vi "SQL查询.vi"(7 "condition":string, 9 "columns":string[](array[string]), 10 "table输入":string(combo), 11 "database":string(combo)) -> (0 "error out":errorcluster, 1 "拆分数据":bool, 2 "columns输出":string[](array[string]), 3 "data":string[][](table))   [LabVIEW 2016, in "数据传输系统-03.lvlib"]
uses:
  <vilib>/Utility/sysdir.llb/System Directory Type.ctl
  <vilib>/addons/database/Connection.llb/DB Tools Open Connec (String).vi
  <vilib>/addons/database/_DB Variant To Data/Database Variant To Data.xnode
  <vilib>/addons/database/NI_Database_API.lvlib
panel:
  out "元素":string
  out "子数组":string[](array[string])
  in  "error in (no error)":errorcluster
  # "时间 > #2021/01/15 08:00:00#and 时间 < #2021/04/15 08:00:00# order by 时间 asc"
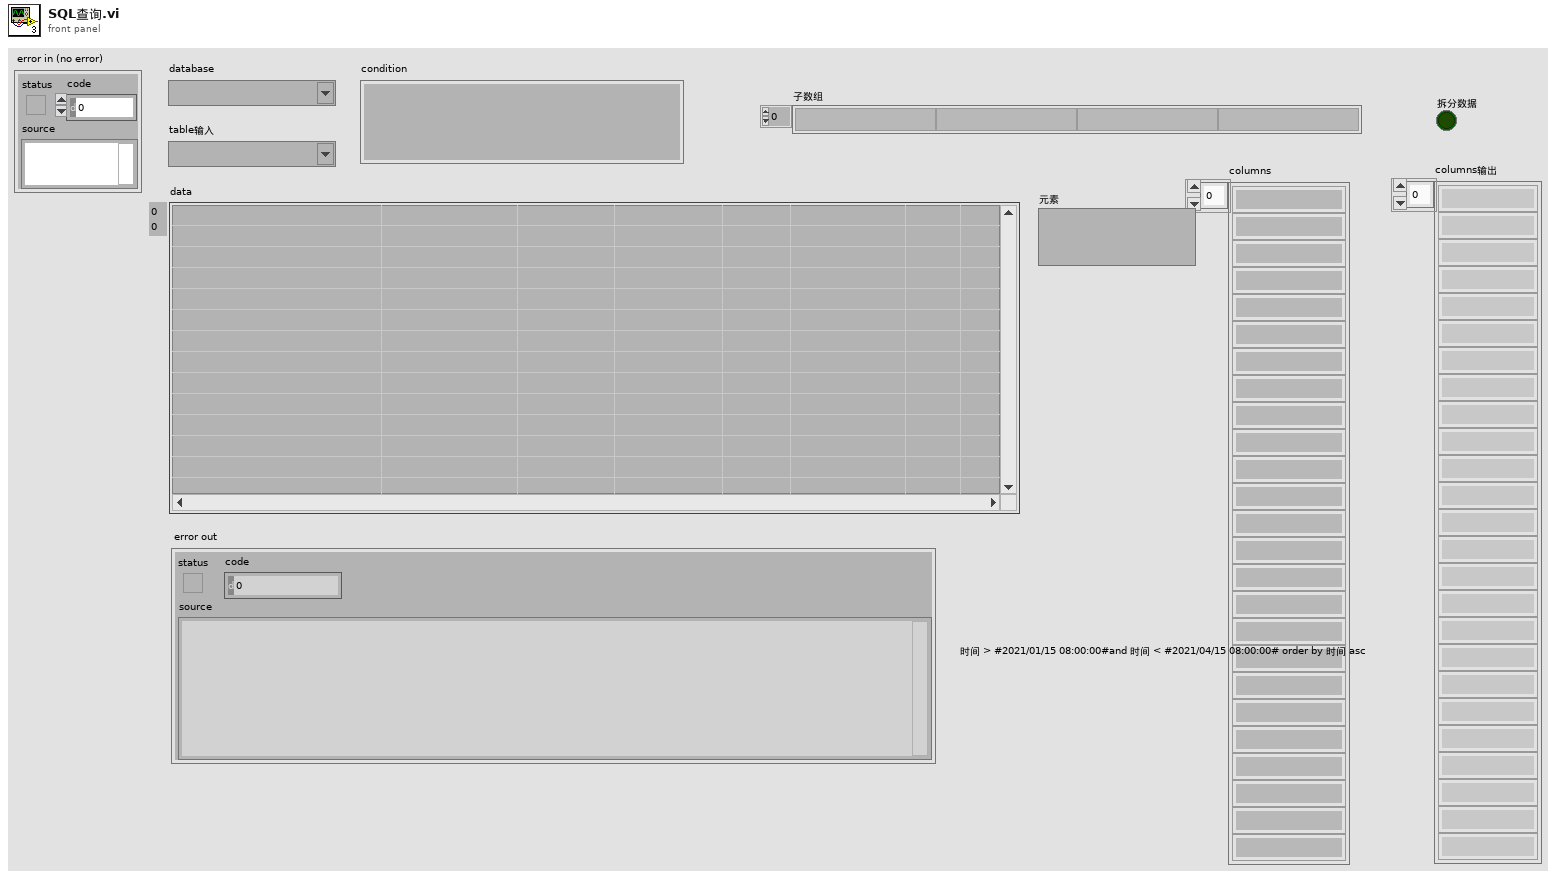
[diagram p1: front panel]
types:
  T1 = typedef "System Directory Type.ctl" = i32
  T2 = typedef "NI_Database_API.lvlib/Conn ObjectReference.ctl" = refnum<k1>
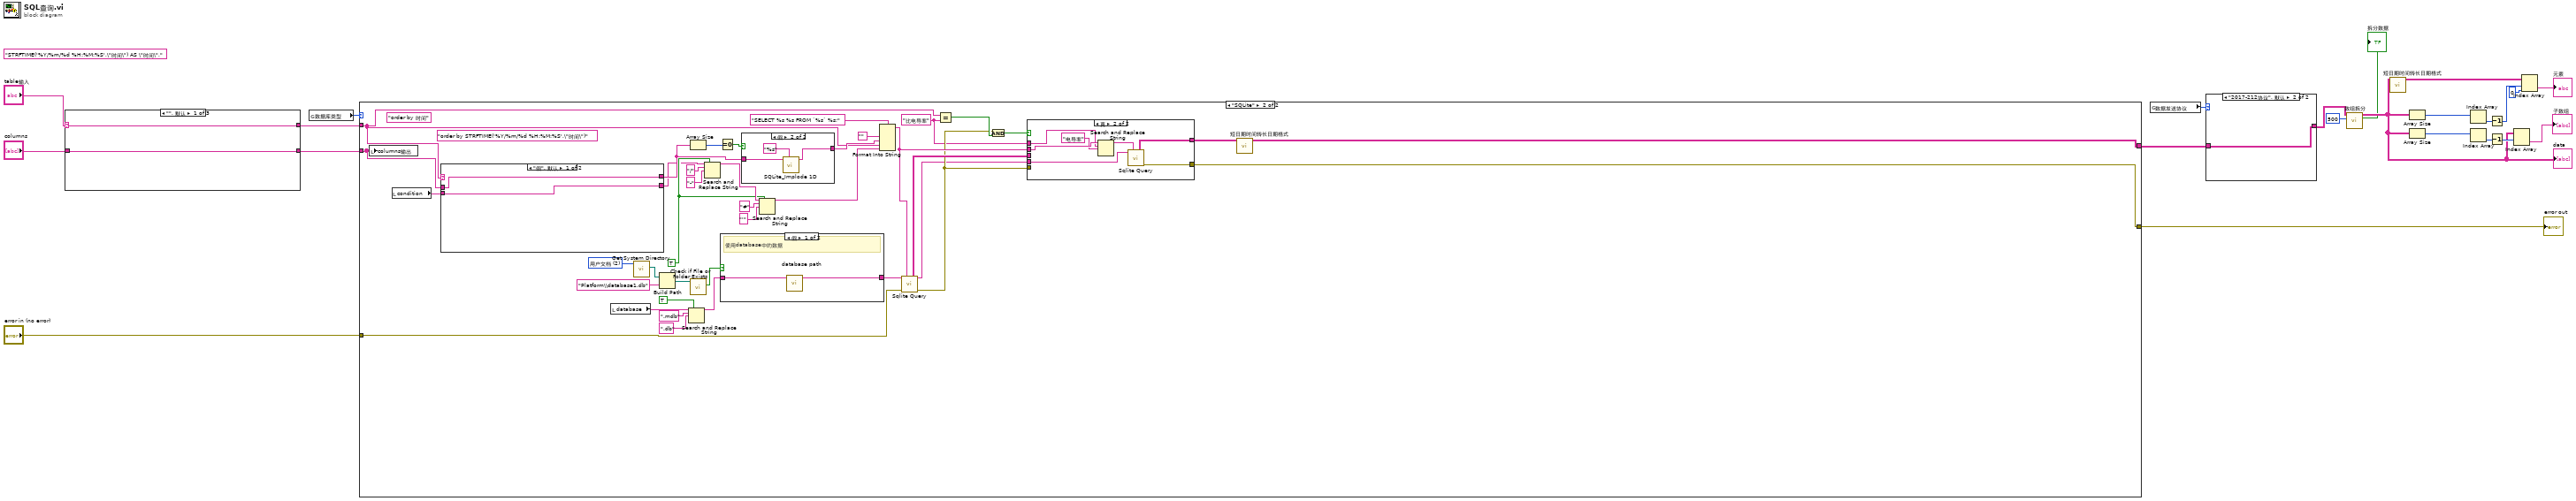
[diagram p0: block diagram]
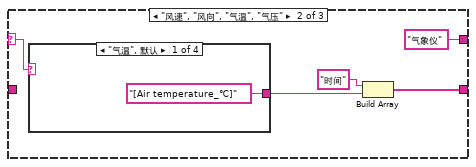
[diagram p2: hidden frame]
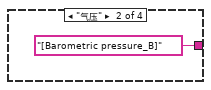
[diagram p3: hidden frame]
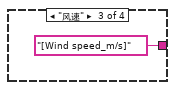
[diagram p4: hidden frame]
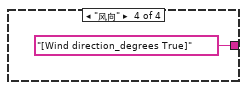
[diagram p5: hidden frame]
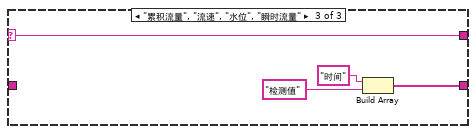
[diagram p6: hidden frame]
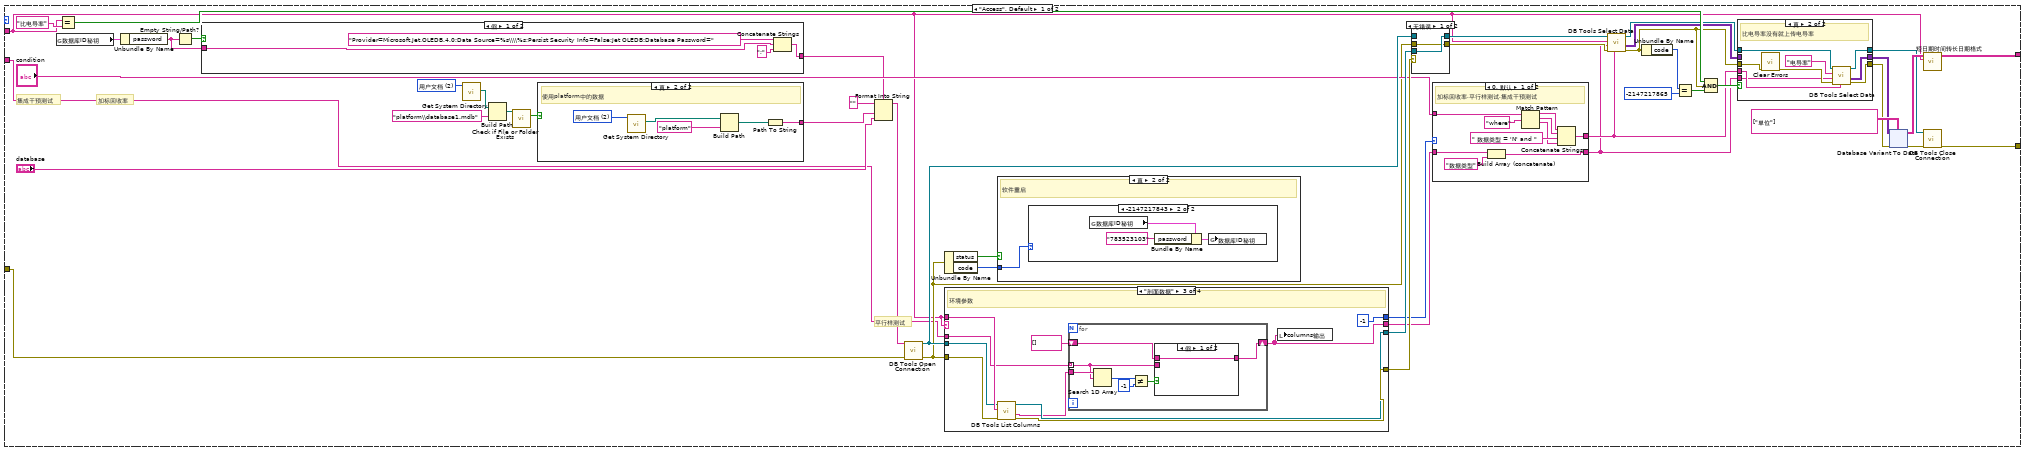
[diagram p7: hidden frame]
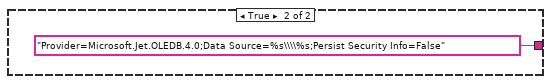
[diagram p8: hidden frame]
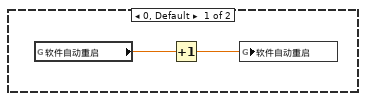
[diagram p10: hidden frame]
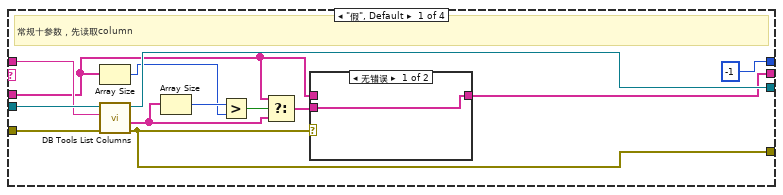
[diagram p13: hidden frame]
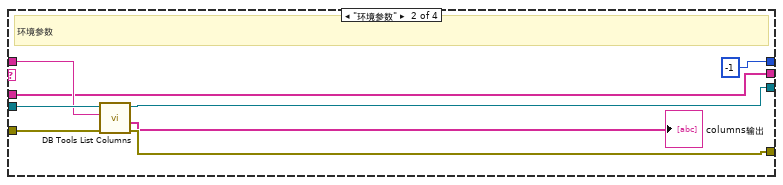
[diagram p15: hidden frame]
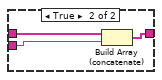
[diagram p16: hidden frame]
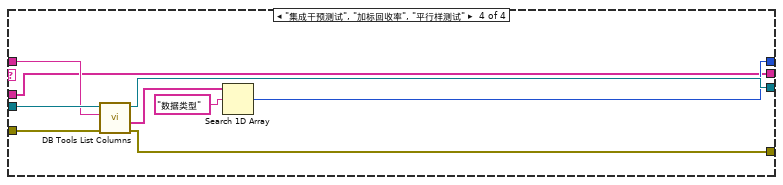
[diagram p17: hidden frame]
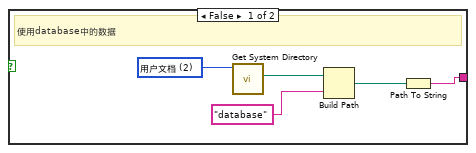
[diagram p19: hidden frame]
diagram:
  (unwired) "STRFTIME('%Y/%m/%d %H:%M:%S',\"时间\") AS \"时间\"," ("输入 1")
  n1 = case shown="\"\", 默认" "table输入" {
    selector: "table输入" -> [w25 w29 w35]
    tunnel: [w25 "气象仪" w35] -> w3
    tunnel: "columns" -> [w24 _ _]
    tunnel: [w24 w26 w37] -> w4
    frame "", Default {
    }
    frame "风速", "风向", "气温", "气压" {
      n2 = case shown="\"气温\", 默认" w29 {
        tunnel: ["[Air temperature_℃]" "[Barometric pressure_B]" "[Wind speed_m/s]" "[Wind direction_degrees True]"] -> w27
        frame "气温", Default {
        }
        frame "气压" {
        }
        frame "风速" {
        }
        frame "风向" {
        }
      }
      n3 = Build Array("时间", w27) -> (w26:string[])
    }
    frame "累积流量", "流速", "水位", "瞬时流量" {
      n4 = Build Array("时间", "检测值") -> (w37:string[])
    }
  }
  n5 = global read "断电保存全局.vi" "数据库类型"() -> (w8:enum16{"Access", "SQLite"})
  n6 = case shown="\"SQLite\"" w8 {
    tunnel: [w79 w264] -> w23
    tunnel: [w51 w240] -> w11
    tunnel: "error in (no error)" -> [w43 w233]
    tunnel: w4 -> [w41 w236]
    tunnel: w3 -> [w40 w235]
    frame "Access", Default {
      w77 = T1 2 items=["用户目录"=0, "用户桌面"=1, "用户文档"=2, "用户应用程序数据"=3, "用户设置"=4, "用户临时目录"=5, "公共文档"=6, "公共应用程序数据"=7, "公共设置"=8, "公共缓存"=13, "系统核心库"=9, "系统安装库"=10, "应用程序文件"=11, "启动盘根目录"=12] ("system directory type")
      # "集成干预测试"
      # "平行样测试"
      # "加标回收率"
      n7 = global read "外部交互全局.vi" "数据库ID秘钥"() -> (w44:cluster{"userID":string, "password":string})
      n8 = Equal?(x=w40, y="比电导率") -> (x = y?=w71:bool)
      n9 = Unbundle By Name(w44) -> ("password"=w45:string)
      n10 = Empty String/Path?(string/path=w45) -> (empty?=w47:bool)
      n11 = case shown="假" w47 {
        tunnel: [w85 "Provider=Microsoft.Jet.OLEDB.4.0;Data Source=%s\\\\%s;Persist Security Info=False" ("格式字符串")] -> w46
        tunnel: w45 -> [w88 _]
        frame False {
          n12 = Concatenate Strings("Provider=Microsoft.Jet.OLEDB.4.0;Data Source=%s\\\\%s;Persist Security Info=False;Jet OLEDB:Database Password=" ("格式字符串"), w88, ";" ("字符串")) -> (w85:string)
        }
        frame True {
        }
      }
      n13 = call <vilib>:"Get System Directory.vi"("system directory type"=w77) -> ("system directory"=w78:path)  [unwired: 10 in]
      n14 = Build Path(base path=w78, name or relative path="platform\\database1.mdb" ("condition")) -> (appended path=w76:path)
      n15 = call <vilib>:"Check if File or Folder Exists.vi"("path"=w76) -> ("file or folder exists?"=w74:bool)  [unwired: 8 in, 2 out]
      n16 = case shown="真" w74 {
        tunnel: [w177 w182] -> w73
        frame False {
          w180 = T1 2 items=["用户目录"=0, "用户桌面"=1, "用户文档"=2, "用户应用程序数据"=3, "用户设置"=4, "用户临时目录"=5, "公共文档"=6, "公共应用程序数据"=7, "公共设置"=8, "公共缓存"=13, "系统核心库"=9, "系统安装库"=10, "应用程序文件"=11, "启动盘根目录"=12] ("system directory type")
          # "使用database中的数据"
          n17 = call <vilib>:"Get System Directory.vi"("system directory type"=w180) -> ("system directory"=w179:path)  [unwired: 10 in]
          n18 = Build Path(base path=w179, name or relative path="database" ("condition")) -> (appended path=w181:path)
          n19 = Path To String(path=w181) -> (string=w177:string)
        }
        frame True {
          w186 = T1 2 items=["用户目录"=0, "用户桌面"=1, "用户文档"=2, "用户应用程序数据"=3, "用户设置"=4, "用户临时目录"=5, "公共文档"=6, "公共应用程序数据"=7, "公共设置"=8, "公共缓存"=13, "系统核心库"=9, "系统安装库"=10, "应用程序文件"=11, "启动盘根目录"=12] ("system directory type")
          # "使用platform中的数据"
          n20 = call <vilib>:"Get System Directory.vi"("system directory type"=w186) -> ("system directory"=w185:path)  [unwired: 10 in]
          n21 = Build Path(base path=w185, name or relative path="platform" ("condition")) -> (appended path=w183:path)
          n22 = Path To String(path=w183) -> (string=w182:string)
        }
      }
      n23 = Format Into String(format string=w46, initial string="" ("初始字符串"), w73, "database") -> (resulting string=w81:string)  [unwired: 1 in, 1 out]
      n24 = call-poly <vilib>:"DB Tools Open Connection.vi"("error in (no error)"=w43, "connection information"=w81) -> ("error out"=w52:errorcluster, "connection reference"=w57:T2)  [unwired: 6 in]
      n25 = Unbundle By Name(w52) -> ("status"=w50:bool, "code"=w39:i32)
      n26 = case shown="\"剖面数据\"" w40 {
        tunnel: w57 -> [w123 w134 w142 w164]
        tunnel: w52 -> [w120 w133 w141 w162]
        tunnel: [w121 w132 w139 w161] -> w59
        tunnel: [w115 w131 w140 w160] -> w60
        tunnel: w40 -> [w122 w130 w143 w163]
        tunnel: [-1 ("index of element") -1 ("index of element") -1 ("index of element") w157] -> w55
        tunnel: w41 -> [w112 w127 w138 w156]
        tunnel: [w113 w127 w135 w156] -> w53
        frame "假", Default {
          # "常规十参数，先读取column"
          n27 = Array Size(array=w112) -> (size(s)=w117:i32)
          n28 = call <vilib>:"DB Tools List Columns.vi"("error in (no error)"=w120, "table"=w122, "connection reference"=w123) -> ("error out"=w115:errorcluster, "columns"=w116:string[], "connection reference out"=w121:T2)  [unwired: 1 in, 1 out]
          n29 = Array Size(array=w116) -> (size(s)=w118:i32)
          n30 = Greater?(x=w118, y=w117) -> (0:w119:bool)
          n31 = Select(t=w112, s=w119, f=w116) -> (s? t:f=w114:string[])
          n32 = case shown="无错误" w115 {
            tunnel: w114 -> [w125 _]
            tunnel: [w125 w126] -> w113
            tunnel: w112 -> [_ w126]
            frame No Error {
            }
            frame Error {
            }
          }
        }
        frame "环境参数" {
          # "环境参数"
          n33 = call <vilib>:"DB Tools List Columns.vi"("error in (no error)"=w133, "table"=w130, "connection reference"=w134) -> ("error out"=w131:errorcluster, "columns"=→"columns输出":string[], "connection reference out"=w132:T2)  [unwired: 1 in, 1 out]
        }
        frame "剖面数据" {
          # "环境参数"
          n34 = call <vilib>:"DB Tools List Columns.vi"("error in (no error)"=w141, "table"=w143, "connection reference"=w142) -> ("error out"=w140:errorcluster, "columns"=w137:string[], "connection reference out"=w139:T2)  [unwired: 1 in, 1 out]
          n35 = for {
            tunnel: w138 -> [w147] mode=indexing
            tunnel: w137 -> [w151]
            shift-right: [w145] -> w135
            shift-left: string[] [] -> [w148]
            n36 = Search 1D Array(1D array=w151, element=w147) -> (index of element=w150:i32)  [unwired: 1 in]
            n37 = Not Equal?(x=w150, y=-1) -> (x != y?=w146:bool)
            n38 = case shown="假" w146 {
              tunnel: w148 -> [w152 w155]
              tunnel: w147 -> [_ w154]
              tunnel: [w152 w153] -> w145
              frame False {
              }
              frame True {
                n39 = Build Array (concatenate)(w155, w154) -> (w153:string[])
              }
            }
          }
          n40 = local write "columns输出"(w135) -> ()
        }
        frame "集成干预测试", "加标回收率", "平行样测试" {
          n41 = call <vilib>:"DB Tools List Columns.vi"("error in (no error)"=w162, "table"=w163, "connection reference"=w164) -> ("error out"=w160:errorcluster, "columns"=w159:string[], "connection reference out"=w161:T2)  [unwired: 1 in, 1 out]
          n42 = Search 1D Array(1D array=w159, element="数据类型" ("元素")) -> (index of element=w157:i32)  [unwired: 1 in]
        }
      }
      n43 = case shown="真" w50 {
        tunnel: w39 -> [_ w90]
        frame False {
        }
        frame True {
          # "软件重启"
          n44 = case shown="-2147217843" w90 {
            frame 0, Default {
              n45 = global read "全局1.vi" "软件自动重启"() -> (w92:dbl)
              n46 = Increment(x=w92) -> (x+1=w91:dbl)
              n47 = global write "全局1.vi" "软件自动重启"(w91) -> ()
            }
            frame -2147217843 {
              n48 = global read "外部交互全局.vi" "数据库ID秘钥"() -> (w93:cluster{"userID":string, "password":string})
              n49 = Bundle By Name(cluster=w93, "password"="783523103") -> (w94:cluster{"userID":string, "password":string})
              n50 = global write "外部交互全局.vi" "数据库ID秘钥"(w94) -> ()
            }
          }
        }
      }
      n51 = case shown="无错误" w60 {
        selector: w60 -> [_ w111]
        tunnel: w59 -> [w109 _]
        tunnel: [w109 w110] -> w58
        tunnel: w57 -> [_ w110]
        tunnel: [w108 w111] -> w56
        tunnel: w52 -> [w108 _]
        frame No Error {
        }
        frame Error {
        }
      }
      n52 = case "条件结构" shown="0, 默认" w55 {
        tunnel: "condition" -> [w103 w106]
        tunnel: w53 -> [w105 w107]
        tunnel: [w97 w107] -> w48
        tunnel: [w96 w106] -> w49
        frame 0, Default {
          # "加标回收率,平行样测试,集成干预测试"
          n53 = Build Array (concatenate)(w105, "数据类型" ("元素")) -> (w97:string[])
          n54 = Match Pattern(string=w103, regular expression="where" ("正则表达式")) -> (before substring=w101:string, match substring=w100:string, after substring=w98:string)  [unwired: 1 in, 1 out]
          n55 = Concatenate Strings(w101, w100, " 数据类型 = 'N' and " ("字符串"), w98) -> (w96:string)
        }
        frame -1 {
        }
      }
      n56 = call <vilib>:"DB Tools Select Data.vi"("condition"=w49, "error in (no error)"=w56, "columns"=w48, "table"=w40, "connection reference"=w58) -> ("error out"=w64:errorcluster, "data"=w66:variant[][], "connection reference out"=w69:T2)  [unwired: 1 in]
      n57 = Unbundle By Name(w64) -> ("code"=w63:i32)
      n58 = Equal?(x=w63, y=-2147217865 ("code")) -> (x = y?=w61:bool)
      n59 = Compound Arithmetic op=AND ("复合运算")(w71, w64, w61) -> (w70:bool)
      n60 = case shown="真" w70 {
        tunnel: w49 -> [_ w176]
        tunnel: w69 -> [w167 w175]
        tunnel: [w167 w170] -> w68
        tunnel: [w166 w171] -> w67
        tunnel: w66 -> [w166 _]
        tunnel: w64 -> [w165 w173]
        tunnel: [w165 w169] -> w65
        tunnel: w48 -> [_ w168]
        frame False {
        }
        frame True {
          # "比电导率没有就上传电导率"
          n61 = call <vilib>:"Clear Errors.vi"("error in (no error)"=w173) -> ("error out"=w172:errorcluster)  [unwired: 5 in, 1 out]
          n62 = call <vilib>:"DB Tools Select Data.vi"("condition"=w176, "error in (no error)"=w172, "columns"=w168, "table"="电导率", "connection reference"=w175) -> ("error out"=w169:errorcluster, "data"=w171:variant[][], "connection reference out"=w170:T2)  [unwired: 1 in]
        }
      }
      n63 = xnode "Database Variant To Data"("database variant"=w67, "error in (no error)"=w65, "type"=string[][] [["单位"]]) -> ("data"=w80:string[][], "error out"=w82:errorcluster)
      n64 = call "短日期时间转长日期格式.vi"("table输入"=w40, "data"=w80) -> ("输出数组"=w79:string[][])  [unwired: 9 in]
      n65 = call <vilib>:"DB Tools Close Connection.vi"("error in (no error)"=w82, "connection reference"=w68) -> ("error out"=w51:errorcluster)  [unwired: 5 in]
    }
    frame "SQLite" {
      w238 = "比电导率" ("y")
      (unwired) "order by STRFTIME('%Y/%m/%d %H:%M:%S',\"时间\")" ("替换字符串(\"\")")
      (unwired) "order by 时间" ("搜索字符串")
      w249 = TRUE ("替换全部？(F)")
      w266 = T1 2 items=["用户目录"=0, "用户桌面"=1, "用户文档"=2, "用户应用程序数据"=3, "用户设置"=4, "用户临时目录"=5, "公共文档"=6, "公共应用程序数据"=7, "公共设置"=8, "公共缓存"=13, "系统核心库"=9, "系统安装库"=10, "应用程序文件"=11, "启动盘根目录"=12] ("system directory type")
      n66 = local write "columns输出"(w236) -> ()
      n67 = local read "condition"() -> (w248:string)
      n68 = case shown="\"假\", 默认" w235 {
        tunnel: w248 -> [w280 w286]
        tunnel: w236 -> [w279 w288]
        tunnel: [w279 w287] -> w259
        tunnel: [w280 w285] -> w247
        frame "假", Default {
        }
        frame "集成干预测试", "加标回收率", "平行样测试" {
          n69 = Build Array (concatenate)(w288, "数据类型" ("元素")) -> (w287:string[])
          n70 = call "数据库加密匹配 (子VI).vi"("输入参数"="N") -> ("Encoded String"=w283:string)  [unwired: 10 in]
          n71 = Match Pattern(string=w286, regular expression="where" ("正则表达式")) -> (before substring=w291:string, match substring=w290:string, after substring=w289:string)  [unwired: 1 in, 1 out]
          n72 = Format Into String(format string=" 数据类型 = '%s' and " ("字符串"), w283) -> (resulting string=w281:string)  [unwired: 2 in, 1 out]
          n73 = Concatenate Strings(w291, w290, w281, w289) -> (w285:string)
        }
      }
      n74 = local read "database"() -> (w251:string)
      n75 = call <vilib>:"Get System Directory.vi"("system directory type"=w266) -> ("system directory"=w265:path)  [unwired: 10 in]
      n76 = Build Path(base path=w265, name or relative path="Platform\\database1.db" ("condition")) -> (appended path=w267:path)
      n77 = Search and Replace String(replace all?=TRUE ("替换全部？(F)"), input string=w251, search string=".mdb" ("搜索字符串"), replace string=".db" ("替换字符串(\"\")")) -> (result string=w246:string)  [unwired: 4 in, 3 out]
      n78 = Array Size(array=w259) -> (size(s)=w263:i32)
      n79 = call <vilib>:"Check if File or Folder Exists.vi"("path"=w267) -> ("file or folder exists?"=w269:bool)  [unwired: 8 in, 2 out]
      n80 = Search and Replace String(replace all?=w249, input string=w247, search string="/" ("搜索字符串"), replace string="-" ("替换字符串(\"\")")) -> (result string=w256:string)  [unwired: 4 in, 3 out]
      n81 = Equal To 0?(x=w263) -> (x = 0?=w262:bool)
      n82 = case shown="假" w269 {
        tunnel: [w299 w300] -> w234
        tunnel: w246 -> [w298 w301]
        frame False {
          # "使用database中的数据"
          n83 = call "database path.vi"("database"=w298) -> ("Path out"=w299:string)  [unwired: 9 in, 1 out]
        }
        frame True {
          # "使用platform中的数据"
          n84 = call "database platform path.vi"("database"=w301) -> ("Path out"=w300:string)  [unwired: 10 in]
        }
      }
      n85 = case shown="假" w262 {
        tunnel: w259 -> [_ w296]
        tunnel: ["*" ("t") w295] -> w260
        frame True {
        }
        frame False {
          n86 = call <userlib>:"SQLite_Implode 1D.vi"("Values"=w296, "format string"="%s") -> ("imploded string"=w295:string)  [unwired: 7 in, 1 out]
        }
      }
      n87 = Search and Replace String(replace all?=w249, input string=w256, search string="#" ("搜索字符串"), replace string="'" ("替换字符串(\"\")")) -> (result string=w231:string)  [unwired: 4 in, 3 out]
      n88 = Format Into String(format string="SELECT %s %s FROM `%s` %s;" ("SQL Query"), "", w260, w235, w231) -> (resulting string=w241:string)  [unwired: 2 in, 1 out]
      n89 = call "Sqlite Query.vi"("DB Path"=w234, "SQL Query"=w241, "error in (no error)"=w233) -> ("Results"=w243:string[][], "DB Path Out"=w237:string, "error out"=w239:errorcluster)  [unwired: 10 in]
      n90 = Equal?(x=w235, y=w238) -> (x = y?=w245:bool)
      n91 = And(x=w239, y=w245) -> (x .and. y?=w244:bool)
      n92 = case shown="真" w244 {
        tunnel: w243 -> [w271 _]
        tunnel: [w271 w278] -> w242
        tunnel: w241 -> [_ w275]
        tunnel: w237 -> [_ w277]
        tunnel: [w270 w276] -> w240
        tunnel: w239 -> [w270 _]
        tunnel: w238 -> [_ w274]
        frame False {
        }
        frame True {
          n93 = Search and Replace String(input string=w275, search string=w274, replace string="电导率" ("Tables Name")) -> (result string=w272:string)  [unwired: 5 in, 3 out]
          n94 = call "Sqlite Query.vi"("DB Path"=w277, "SQL Query"=w272) -> ("Results"=w278:string[][], "error out"=w276:errorcluster)  [unwired: 11 in, 1 out]
        }
      }
      n95 = call "短日期时间转长日期格式.vi"("data"=w242) -> ("输出数组"=w264:string[][])  [unwired: 10 in]
    }
  }
  "error out" <- w11
  n96 = global read "断电保存全局.vi" "数据发送协议"() -> (w22:enum16{"2005-212协议", "2017-212协议"})
  n97 = case shown="\"2017-212协议\", 默认" w22 {
    tunnel: w23 -> [w303 w310]
    tunnel: [w302 w310] -> w9
    frame "2005-212协议" {
      n98 = for {
        N: 1 -> [_]
        tunnel: string[][] [] ("data") -> [w309]
        tunnel: w303 -> [w308] mode=indexing
        tunnel: [w306] -> w302
        n99 = Insert Into Array(array=w309, index (row)=0 ("索引 (行)"), new element=w308) -> (w306:string[][])  [unwired: 1 in]
      }
    }
    frame "2017-212协议", Default {
    }
  }
  n100 = call "数组拆分.vi"("拆分大小"=500, "输入数据"=w9) -> ("拆分数据"=→"拆分数据":bool, "输出数组"=w2:string[][])  [unwired: 8 in]
  "data" <- w2
  n101 = call "短日期时间转长日期格式.vi"("data"=w2) -> ("输出数组"=w17:string[][])  [unwired: 10 in]
  n102 = Array Size(array=w2) -> (size(s)=w16:i32[])
  n103 = Array Size(array=w2) -> (size(s)=w21:i32[])
  n104 = Index Array(array=w16) -> (element=w15:i32)  [unwired: 1 in]
  n105 = Index Array(array=w21) -> (element=w19:i32)  [unwired: 1 in]
  n106 = Decrement(x=w15) -> (x-1=w14:i32)
  n107 = Decrement(x=w19) -> (x-1=w18:i32)
  n108 = Index Array(array=w2, index (row)=w18) -> (element=→"子数组":string[])  [unwired: 1 in]
  n109 = Index Array(array=w17, index (row)=w14, index (col)=0 ("禁用的索引 (列)")) -> (element=→"元素":string)
